vi "Simple Add.vi"(9 "Addend 3":dbl format="%#_13g", 10 "Addend 2":dbl format="%#_13g", 11 "Addend 1":dbl format="%#_13g") -> (3 "Sum":dbl)   [LabVIEW 2015]
panel:
  in  "Addend 4":dbl format="%#_13g"
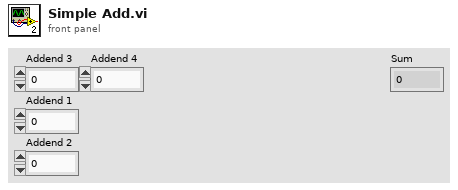
[diagram p1: front panel]
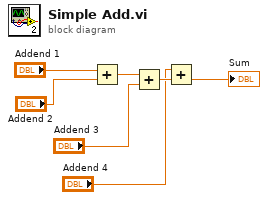
[diagram p0: block diagram]
diagram:
  n1 = Add(x="Addend 1", y="Addend 2") -> (x+y=w5:dbl)
  n2 = Add(x=w5, y="Addend 3") -> (x+y=w3:dbl)
  n3 = Add(x="Addend 4", y=w3) -> (x+y=→"Sum":dbl)
